vi "getData.vi"() -> ()   [LabVIEW 2010]
panel:
  in  "mode (0)":i16
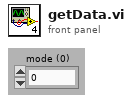
[diagram p1: front panel]
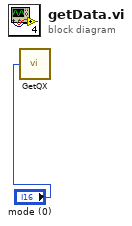
[diagram p0: block diagram]
diagram:
  n1 = call "GetQX.vi"("mode (0)"="mode (0)") -> ()
